vi "Contador.vi"() -> ()   [LabVIEW 2010]
panel:
  in  "Parar SubVI":bool
  out "Loop2":bool
  out "Iteracion":i32
  in  "Inicio":i32
  out "Incrementa":i32
  out "Decrementa":i32
  out "Loop1":bool
  in  "stop":bool=TRUE
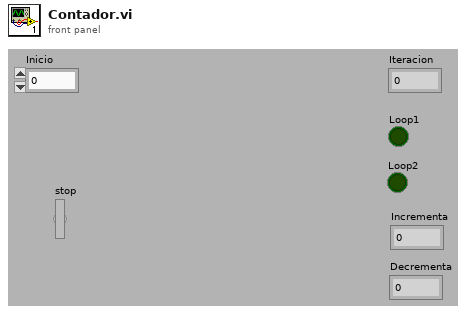
[diagram p1: front panel]
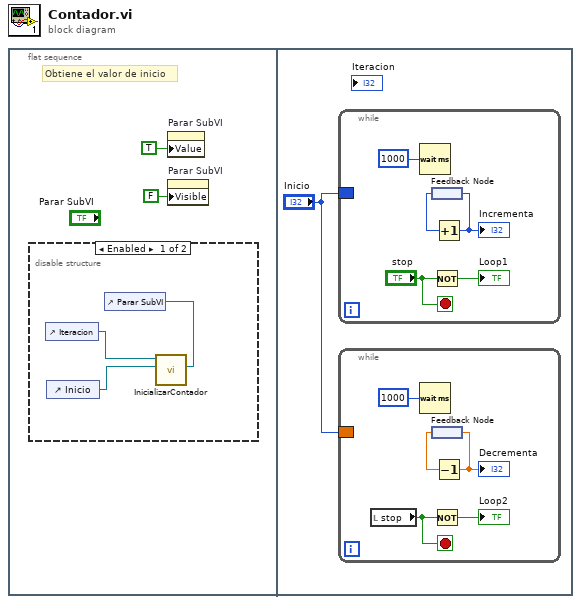
[diagram p0: block diagram]
diagram:
  n1 = flat-sequence {
    frame #0 {
      # "Obtiene el valor de inicio"
      n2 = disable-structure shown="Enabled" {
        frame Enabled {
          n3 = control-ref of="Iteracion"() -> (w5:refnum<vi>)
          n4 = control-ref of="Inicio"() -> (w4:refnum<vi>)
          n5 = control-ref of="Parar SubVI"() -> (w3:refnum<vi>)
          n6 = call "InicializarContador.vi"("stop 2"=w3, "Incio"=w4, "Iteracion"=w5) -> ()  [unwired: 9 in]
        }
        frame Disabled {
        }
      }
      n7 = property on="Parar SubVI" class="Bool (strict)"("Value"=TRUE ("Parar SubVI")) -> ()  [unwired: 2 in, 2 out]
      n8 = property on="Parar SubVI" class="Bool (strict)"("Visible"=FALSE) -> ()  [unwired: 2 in, 2 out]
    }
    frame #1 {
      n9 = while {
        border: "Inicio" -> [_]
        stop <- "stop" stop-if-true
        n10 = Wait (ms)(milliseconds to wait=u32 1000) -> ()  [unwired: 1 out]
        n11 = feedback #1() -> (w14:i32)
        n12 = Not(x="stop") -> (.not. x?=→"Loop1":bool)
        n13 = Increment(x=w14) -> (x+1=w15:i32)
        "Incrementa" <- w15
        n14 = feedback-in #1(w15) -> ()
      }
      n15 = while {
        border: "Inicio" -> [_]
        stop <- w7 stop-if-true
        n16 = local read "stop"() -> (w7:bool)
        n17 = Wait (ms)(milliseconds to wait=u32 1000) -> ()  [unwired: 1 out]
        n18 = feedback #2() -> (w9:dbl)
        n19 = Not(x=w7) -> (.not. x?=→"Loop2":bool)
        n20 = Decrement(x=w9) -> (x-1=w10:dbl)
        "Decrementa" <- w10
        n21 = feedback-in #2(w10) -> ()
      }
    }
  }
